vi "emi_Dialog End.vi"(11 "error in":errorcluster) -> (15 "error out":errorcluster)   [LabVIEW 2011]
doc: "Closes the dialog box, setting behavior back to default"
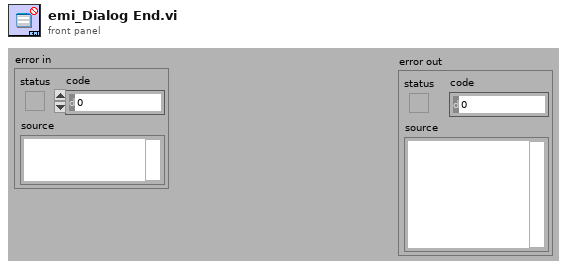
[diagram p1: front panel]
types:
  T1 = enum32{"Invalid", "Default", "Floating", "Floating/Auto-Hide", "Modal"}
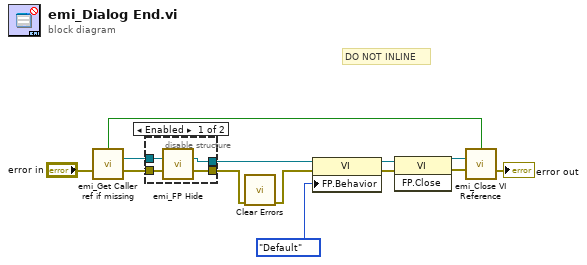
[diagram p0: block diagram]
diagram:
  # "DO NOT INLINE"
  n1 = call "emi_Get Caller ref if missing.vi"("error in (no error)"="error in") -> ("Ref Generated"=w3:bool, "VI Refnum Out"=w12:refnum<vi>, "error out"=w11:errorcluster)  [unwired: 12 in]
  n2 = disable-structure shown="Enabled" {
    disable-tunnel: w12 -> [w17 w19]
    disable-tunnel: w11 -> [w16 w18]
    disable-tunnel: [w15 w19] -> w5
    disable-tunnel: [w14 w18] -> w2
    frame Enabled {
      n3 = call "emi_FP Hide.vi"("VI Refnum(This vi)"=w17, "error in (no error)"=w16) -> ("VI Refnum"=w15:refnum<vi>, "error out"=w14:errorcluster)  [unwired: 12 in]
    }
    frame Disabled {
    }
  }
  n4 = call <vilib>:"Clear Errors.vi"("error in (no error)"=w2) -> ("error out"=w1:errorcluster)  [unwired: 6 in]
  n5 = property class="VI"(reference=w5, error in=w1, "FP.Behavior"=T1."Default" ("Front Panel Window:Behavior")) -> (reference out=w6:refnum<vi>, error out=w7:errorcluster)
  n6 = invoke class="VI" method="FP.Close"(reference=w6, error in=w7) -> (reference out=w4:refnum<vi>, error out=w8:errorcluster)  [unwired: 1 in, 1 out]
  n7 = call "emi_Close VI Reference.vi"("Close ref?(T)"=w3, "VI Refnum"=w4, "error in (no error)"=w8) -> ("error out"=→"error out":errorcluster)  [unwired: 11 in, 1 out]
